vi "CheckRTMasterLoop.vi"(8 "error in (no error)":errorcluster) -> (0 "error out":errorcluster, 2 "CAlexVersion":T1, 3 "RTMasterLoopRunning":bool)   [LabVIEW 2016]
uses:
  Classes/CAlex2/TypeDef/CAlexVersion.ctl
  Classes/CAlex2/CAlex2.lvclass
panel:
  in  "Cancel Button":bool
  in  "OK Button":bool
  # "Please run RT Master Loop VI"
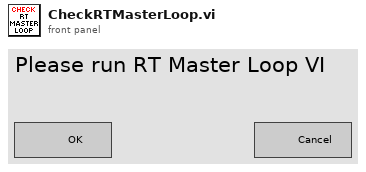
[diagram p1: front panel]
types:
  T1 = typedef "CAlex2.lvclass/CAlexVersion.ctl" = enum16{"Mobile", "MobileLeft\n", "Treadmill", "Treadmill Left\n"}
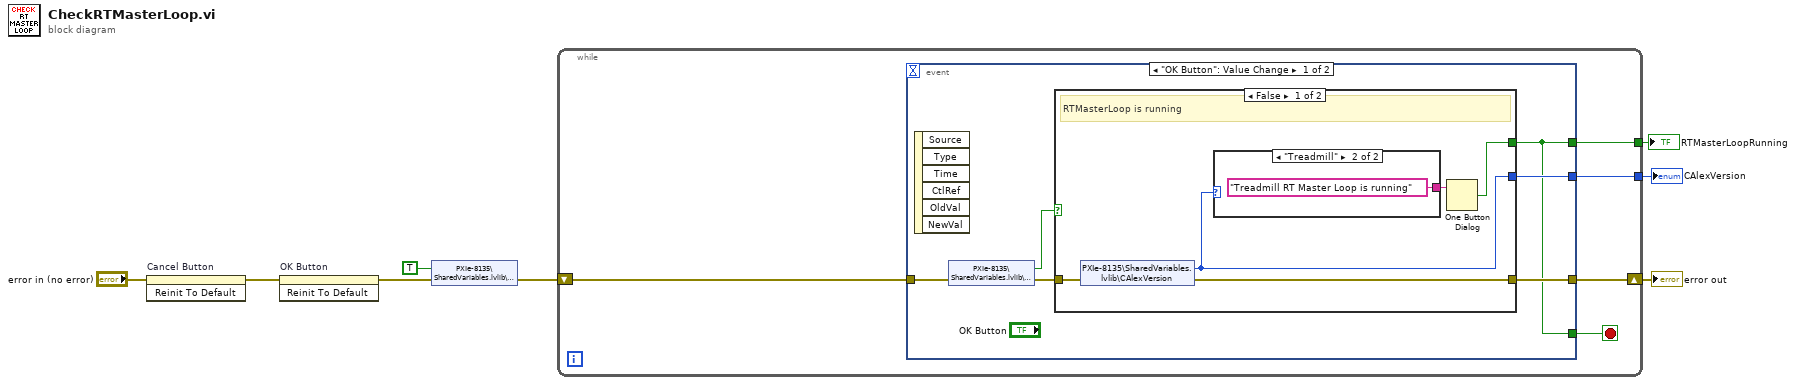
[diagram p0: block diagram]
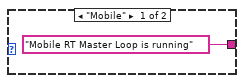
[diagram p2: hidden frame]
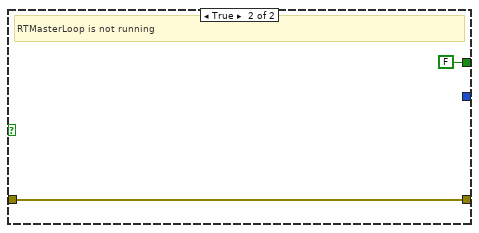
[diagram p3: hidden frame]
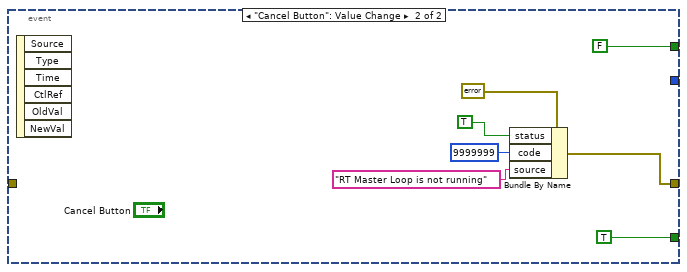
[diagram p4: hidden frame]
diagram:
  n1 = invoke on="Cancel Button" class="Bool" method="Reinit To Default"(error in="error in (no error)") -> (error out=w3:errorcluster)  [unwired: 2 in, 2 out]
  n2 = invoke on="OK Button" class="Bool" method="Reinit To Default"(error in=w3) -> (error out=w2:errorcluster)  [unwired: 2 in, 2 out]
  n3 = shared-variable "PXIe-8135\\SharedVariables.lvlib\\Stop RT"(TRUE ("GlobalStop"), error in=w2) -> (error out=w7:errorcluster)
  n4 = while {
    shift-right: [w13] -> w8
    shift-left: w7 -> [w10]
    tunnel: [w9] -> w5
    tunnel: [w11] -> w4
    stop <- w12 stop-if-true
    n5 = event shown="[0] \"OK Button\": Value Change" {
      selector: _ -> [_ _]
      dyn-events: _ -> [_ _]
      timeout: _ -> [_ _]
      tunnel: [w19 w31] -> w13
      tunnel: [w14 TRUE] -> w12
      tunnel: [w18 _] -> w11
      tunnel: w10 -> [w17 _]
      tunnel: [w14 FALSE ("true")] -> w9
      event "OK Button": Value Change {
        n6 = event-data() -> ()  [unwired: 1 in, 6 out]
        n7 = shared-variable "PXIe-8135\\SharedVariables.lvlib\\Stop RT"(error in=w17) -> (w15:bool, error out=w16:errorcluster)
        n8 = case shown="False" w15 {
          tunnel: w16 -> [w24 w28]
          tunnel: [w23 w28] -> w19
          tunnel: [w22 _] -> w18
          tunnel: [w21 FALSE ("true")] -> w14
          frame False {
            # "RTMasterLoop is running"
            n9 = shared-variable "PXIe-8135\\SharedVariables.lvlib\\CAlexVersion"(error in=w24) -> (w22:T1, error out=w23:errorcluster)
            n10 = case shown="\"Treadmill\"" w22 {
              tunnel: ["Mobile RT Master Loop is running" "Treadmill RT Master Loop is running"] -> w20
              frame "Mobile" {
              }
              frame "Treadmill" {
              }
            }
            n11 = One Button Dialog(message=w20) -> (true=w21:bool)  [unwired: 1 in]
          }
          frame True {
            # "RTMasterLoop is not running"
          }
        }
      }
      event "Cancel Button": Value Change {
        n12 = event-data() -> ()  [unwired: 1 in, 6 out]
        n13 = Bundle By Name(cluster=errorcluster {"status"=FALSE, "code"=0, "source"=""} ("error in (no error)"), "status"=TRUE, "code"=9999999, "source"="RT Master Loop is not running") -> (w31:errorcluster)
      }
    }
  }
  "error out" <- w8
  "RTMasterLoopRunning" <- w5
  "CAlexVersion" <- w4
